vi "Assert Almost Equal_Float.vi"(3 "Execution time (s)":dbl=-1.0, 4 "Use Percentage of X (F)":bool, 5 "Assert Only? (F)":bool, 6 "error code (1)":i32=1, 7 "Label":string, 8 "error in (no error)":errorcluster, 9 "Tolerance":ext=0.00000100000000000000000004, 10 "Y":ext, 11 "X":ext) -> (0 "error out":errorcluster)   [LabVIEW 2013, in "Caraya.lvlib" / "Assert.lvclass"]
doc: "Generates an error if the input condition is not met.\n\nTolerance is either an absolute or percentage value, depending on the \"Use Percentage of X\" flag. Defaults to absolute, tolerance = 1E-6.\nWhen Percentage mode, percentage is calculated based on value of X.\n\n\n--\nCopyright © 2015 JKI All rights reserved.\n\nAuthor: Tomi Maila <tomi.maila@jki.net>\n\nThis library is provided \"AS IS\" ,WITHOUT WARRANTIES OR\nCONDITIONS OF ANY KIND, either express or implied.\n\nJKI -- jki.net"
uses:
  Assert.lvclass
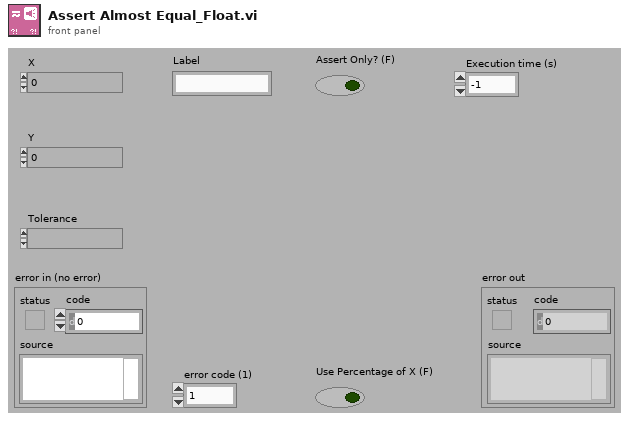
[diagram p1: front panel]
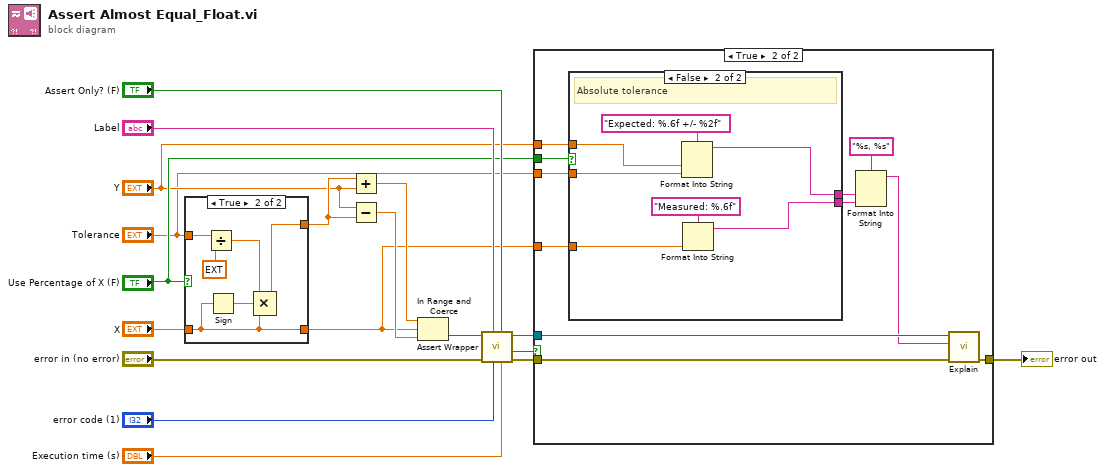
[diagram p0: block diagram]
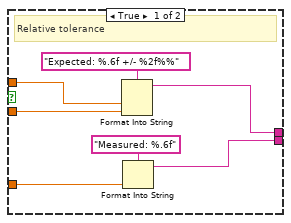
[diagram p3: hidden frame]
diagram:
  n1 = case shown="True" "Use Percentage of X (F)" {
    tunnel: "Tolerance" -> [w20 w26]
    tunnel: [w20 w23] -> w11
    tunnel: "X" -> [w19 w22]
    tunnel: [w19 w22] -> w6
    frame False {
    }
    frame True {
      n2 = Divide(x=w26, y=ext 100.0) -> (x/y=w21:ext)
      n3 = Sign(1:w22) -> (0:w24:ext)
      n4 = Compound Arithmetic op=MULTIPLY(w21, w24, w22) -> (w23:ext)
    }
  }
  n5 = Add(x=w11, y="Y") -> (x+y=w13:ext)
  n6 = Subtract(x="Y", y=w11) -> (x-y=w12:ext)
  n7 = In Range and Coerce(upper limit=w13, x=w6, lower limit=w12) -> (In Range?=w15:bool)  [unwired: 1 out]
  n8 = call "Assert Wrapper.vi"("Execution time (s)"="Execution time (s)", "Assert Only? (F)"="Assert Only? (F)", "error code (1)"="error code (1)", "Label"="Label", "error in (no error)"="error in (no error)", "Assert?"=w15) -> ("error out"=w2:errorcluster, "Verbose"=w3:bool, "Assert out"=w1:refnum<class "Assert.lvclass">)  [unwired: 3 in]
  n9 = case shown="True" w3 {
    tunnel: [w27 w38] -> w9
    tunnel: w1 -> [_ w37]
    tunnel: w2 -> [w27 w36]
    tunnel: "Use Percentage of X (F)" -> [_ w32]
    tunnel: "Y" -> [_ w31]
    tunnel: w6 -> [_ w30]
    tunnel: "Tolerance" -> [_ w29]
    frame False {
    }
    frame True {
      n10 = case shown="False" w32 {
        tunnel: [w44 w51] -> w34
        tunnel: [w42 w49] -> w33
        tunnel: w31 -> [w40 w47]
        tunnel: w30 -> [w41 w48]
        tunnel: w29 -> [w39 w46]
        frame True {
          # "Relative tolerance"
          n11 = Format Into String(format string="Expected: %.6f +/- %2f%%", w40, w39) -> (resulting string=w44:string)  [unwired: 2 in, 1 out]
          n12 = Format Into String(format string="Measured: %.6f", w41) -> (resulting string=w42:string)  [unwired: 2 in, 1 out]
        }
        frame False {
          # "Absolute tolerance"
          n13 = Format Into String(format string="Expected: %.6f +/- %2f", w47, w46) -> (resulting string=w51:string)  [unwired: 2 in, 1 out]
          n14 = Format Into String(format string="Measured: %.6f", w48) -> (resulting string=w49:string)  [unwired: 2 in, 1 out]
        }
      }
      n15 = Format Into String(format string="%s, %s", w34, w33) -> (resulting string=w28:string)  [unwired: 2 in, 1 out]
      n16 = call "Explain.vi"("error in (no error)"=w36, "Verbose Explanation"=w28, "Assert in"=w37) -> ("error out"=w38:errorcluster)  [unwired: 7 in, 1 out]
    }
  }
  "error out" <- w9
